vi "Open All Shared Variables for Write Access.vi"(8 "error in":errorcluster, 11 "Variable Names":string[](array[string])) -> (0 "error out":errorcluster, 3 "Shared Variable Connections":refnum<k21>[](array[refnum]))   [LabVIEW 2017, in "DTACQ - Network Enabled Device Driver.lvlib"]
uses:
  DTACQ - Network Enabled Device Driver.lvlib
  Network Shared Variables/Typedefs/X and Y Variant Arrays--Cluster.ctl
  Network Shared Variables/Shared Variables Library.lvlib
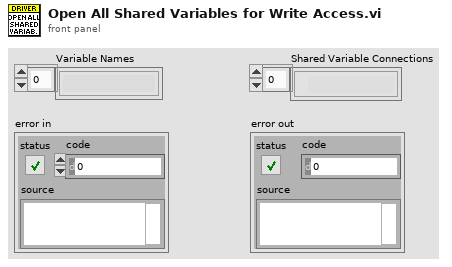
[diagram p1: front panel]
types:
  T1 = cluster{"Read Access":enum8{"Allowed", "Required", "Denied"}, "Write Access":enum8{"Allowed", "Required", "Denied"}}
  T2 = cluster{"Read Access":enum8{"Allowed", "Required", "None"}, "Write Access":enum8{"Allowed", "Required", "None"}}
  T3 = typedef "Shared Variables Library.lvlib/X and Y Variant Arrays--Cluster.ctl" = cluster{"X-Data":variant[], "Y-Data":variant[]}
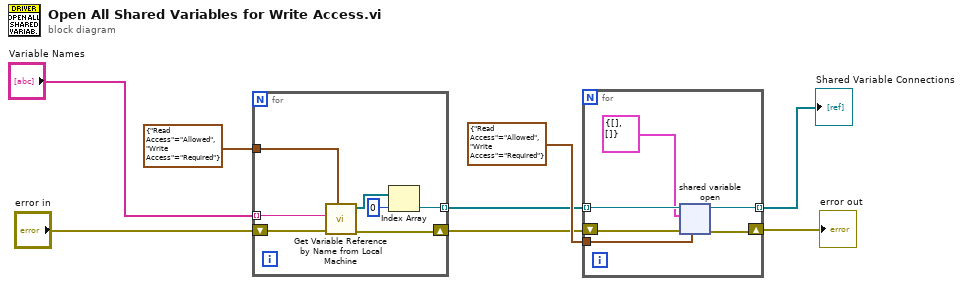
[diagram p0: block diagram]
diagram:
  n1 = for {
    shift-right: [w13] -> w5
    shift-left: "error in" -> [w15]
    tunnel: "Variable Names" -> [w14] mode=indexing
    tunnel: [w12] -> w4 mode=indexing
    tunnel: T1 {"Read Access"=enum."Allowed", "Write Access"=enum."Required"} ("Access Type") -> [w9]
    n2 = call "Get Variable Reference by Name from Local Machine.vi"("Access Type"=w9, "error in"=w15, "Search"=w14) -> ("error out"=w13:errorcluster, "Variable References Out"=w11:refnum<k21>[])  [unwired: 6 in, 1 out]
    n3 = Index Array(array=w11, index=0) -> (element=w12:refnum<k21>)
  }
  n4 = for {
    tunnel: w4 -> [w21] mode=indexing
    tunnel: [w18] -> w8 mode=indexing
    tunnel: T2 {"Read Access"=enum."Allowed", "Write Access"=enum."Required"} ("access") -> [w16]
    shift-right: [w17] -> w1
    shift-left: w5 -> [w20]
    n5 = shared-variable-open(w21, w20, T3 {"X-Data"=[], "Y-Data"=[]} ("Data Cluster"), w16) -> (w18:refnum<k21>, w17:errorcluster)
  }
  "Shared Variable Connections" <- w8
  "error out" <- w1
